vi "RH_PPMU_Set0A.vi"(8 "error in":errorcluster, 9 "Settling (s)":dbl, 10 "channel list":string, 11 "PPMU Session In":refnum<k15>) -> (0 "error out":errorcluster, 3 "PPMU Session Out":refnum<k15>)   [LabVIEW 2023, in "ResourceHandling.lvlib"]
doc: "Set 0A, start sourcing and waits a settling time"
uses:
  ResourceHandling.lvlib
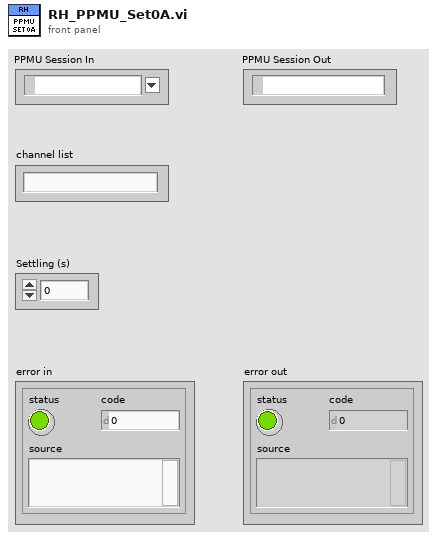
[diagram p1: front panel]
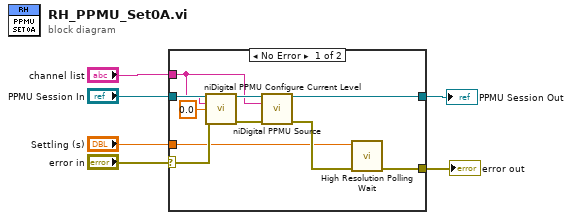
[diagram p0: block diagram]
diagram:
  n1 = case shown="No Error" "error in" {
    selector: "error in" -> [w10 w17]
    tunnel: "PPMU Session In" -> [w16 w18]
    tunnel: "channel list" -> [w12 _]
    tunnel: [w8 w17] -> w3
    tunnel: [w11 w18] -> w4
    tunnel: "Settling (s)" -> [w7 _]
    frame No Error {
      n2 = call <instrlib>:"niDigital PPMU Configure Current Level.vi"("instrument handle"=w16, "channel list"=w12, "current level (A)"=0.0 ("voltage level (V)"), "error in"=w10) -> ("instrument handle out"=w14:refnum<k15>, "error out"=w13:errorcluster)  [unwired: 10 in]
      n3 = call <instrlib>:"niDigital PPMU Source.vi"("instrument handle"=w14, "channel list"=w12, "error in"=w13) -> ("instrument handle out"=w11:refnum<k15>, "error out"=w9:errorcluster)  [unwired: 11 in]
      n4 = call <vilib>:"High Resolution Polling Wait.vi"("error in (no error)"=w9, "seconds to wait"=w7) -> ("error out"=w8:errorcluster)  [unwired: 9 in]
    }
    frame Error {
    }
  }
  "error out" <- w3
  "PPMU Session Out" <- w4
